vi "Move to Index.vi"(11 "index":i32) -> (3 "Image Value":i32)   [LabVIEW 2018]
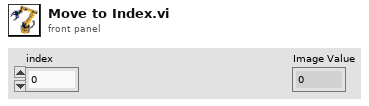
[diagram p1: front panel]
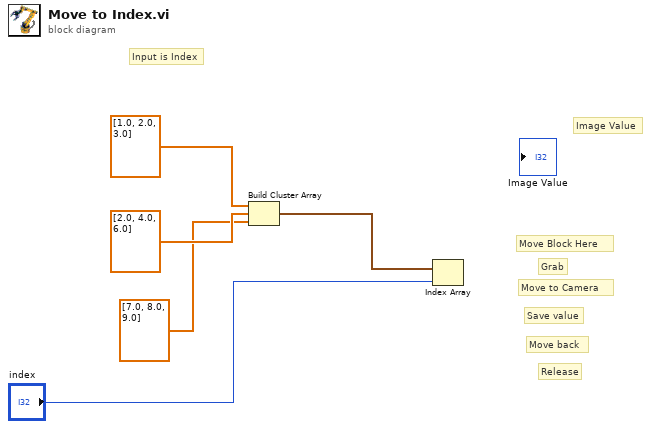
[diagram p0: block diagram]
diagram:
  # "Image Value"
  # "Release"
  # "Move back"
  # "Save value"
  # "Move to Camera"
  # "Grab"
  # "Move Block Here"
  # "Input is Index"
  n1 = Build Cluster Array(dbl[] [1.0, 2.0, 3.0], dbl[] [2.0, 4.0, 6.0], dbl[] [7.0, 8.0, 9.0]) -> (w2:cluster{dbl, dbl, dbl}[])
  n2 = Index Array(array=w2, index="index") -> ()  [unwired: 1 out]
